vi "Read Setup File Name.vi"(8 "error in (no error)":errorcluster, 11 "VISA resource name":refnum<visa-resource-name>) -> (0 "error out":errorcluster, 2 "Setup File":string, 3 "VISA resource name out":refnum<visa-resource-name>)   [LabVIEW 2010, in "Temptronic TP04300.lvlib"]
doc: "This VI reads the name of the test setup file currently in use."
uses:
  Temptronic TP04300.lvlib
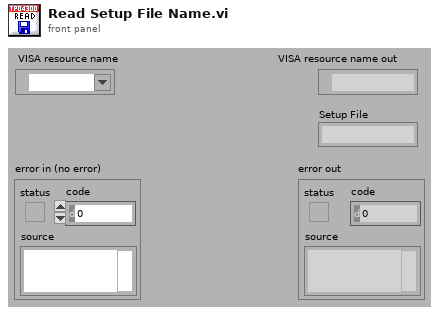
[diagram p1: front panel]
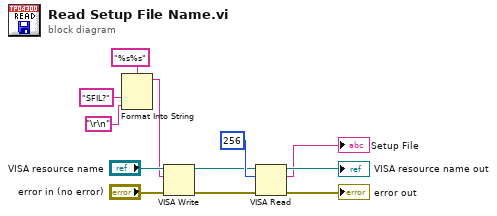
[diagram p0: block diagram]
diagram:
  n1 = Format Into String(format string="%s%s", "SFIL?" ("format string"), "\r\n") -> (resulting string=w4:string)  [unwired: 2 in, 1 out]
  n2 = VISA Write(VISA resource name="VISA resource name", write buffer=w4, error in (no error)="error in (no error)") -> (VISA resource name out=w1:refnum<visa-resource-name>, error out=w2:errorcluster)  [unwired: 1 out]
  n3 = VISA Read(VISA resource name=w1, byte count=u32 256, error in (no error)=w2) -> (VISA resource name out=→"VISA resource name out":refnum<visa-resource-name>, read buffer=→"Setup File":string, error out=→"error out":errorcluster)  [unwired: 1 out]
